vi "GlobalTest.vi"() -> ()   [LabVIEW 2019]
uses:
  TypeDefs/AcqMode.ctl
panel:
  in  "Comment":string
  in  "Temperature (K)":dbl=5.0 caption="T ="
  out "Excitation Power (uW)":dbl=0.2 caption="P    =" format="%#_3p"
  in  "Excitation Source":enum16{"P", "CW", "SK"}(ring)=enum."CW" caption="Laser"
  in  "Acq Time (ms)":dbl=100.0 caption="T" min=1.0 max=360000.0 step=50.0
  in  "Acq Mode":T1=enum."Spectrum" caption="Mode :"
  in  "Experiment Name":string="B1802CF_QD0"
  # "exc"
  # "W"
  # "ms"
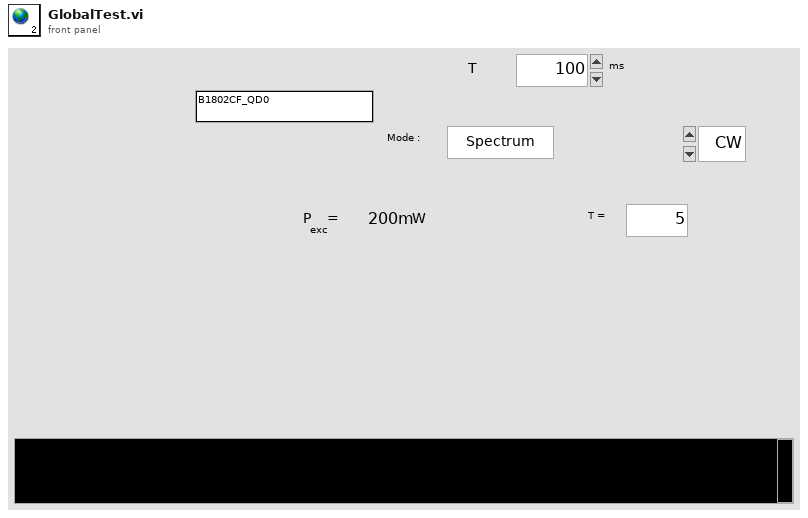
[diagram p1: front panel]
types:
  T1 = typedef "AcqMode.ctl" = enum16{"Image", "Spectrum", "APD 1", "APD 2", "APD 1+2"}
diagram:
